vi "FakeSendCommand.vi"(8 "error in (no error)":errorcluster, 10 "Enum":enum16{"Push", "Pull", "Pause"}(ring), 11 "VISA resource name":refnum<visa-resource-name>) -> (0 "error out":errorcluster, 1 "FakeError":bool, 2 "Response":enum16{"Push", "Pull", "Pause"}(ring), 3 "VISA resource name out":refnum<visa-resource-name>)   [LabVIEW 2018]
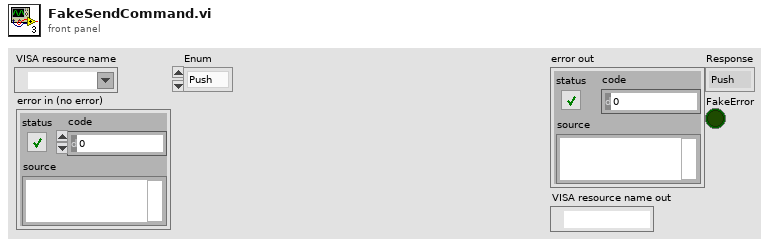
[diagram p1: front panel]
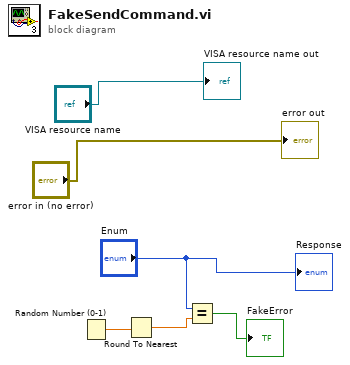
[diagram p0: block diagram]
diagram:
  n1 = Random Number (0-1)() -> (number: 0 to 1=w4:dbl)
  n2 = Round To Nearest(number=w4) -> (nearest integer value=w3:dbl)
  n3 = Equal?(x="Enum", y=w3) -> (x = y?=→"FakeError":bool)
  "VISA resource name out" <- "VISA resource name"
  "error out" <- "error in (no error)"
  "Response" <- "Enum"
